vi "test_json.vi"() -> ()   [LabVIEW 2019, in "Inst.Krohn-Hite-7008.lvclass"]
uses:
  Inst.Krohn-Hite-7008.lvclass
  KH7008/typedefs/allChannelProperties--Array.ctl
  KH7008/typedefs/channelProperties--Cluster.ctl
  KH7008/typedefs/channel--enum.ctl
  KH7008/typedefs/gain--enum.ctl
  KH7008/typedefs/Input--Enum.ctl
  KH7008/typedefs/shunt--enum.ctl
  KH7008/typedefs/couple--Enum.ctl
  KH7008/typedefs/Filter--Enum.ctl
  Typedefs/setAllChannelsRequest--Cluster.ctl
  aca3e566-98a3-49c5-b33f-164d3aa1c4d2.vi
  <vilib>/JDP Science/JSONtext/Variant to JSON Text.vi
  <vilib>/addons/_JKI Toolkits/Caraya/classes/Assert/Assert Equal Value and Type_Variant.vi
  <vilib>/JDP Science/JSONtext/LVClass Serializer/JSONtext LVClass Serializer.lvclass
  KH7008/KH7008.lvlib
  <vilib>/JDP Science/JSONtext/JSONtext.lvlib
  <vilib>/addons/_JKI Toolkits/Caraya/classes/Assert/Assert.lvclass
  <vilib>/addons/_JKI Toolkits/Caraya/classes/Test/Test.lvclass
panel:
  out "allChannelProperties":T1
  in  "Channel Parameters out":T1
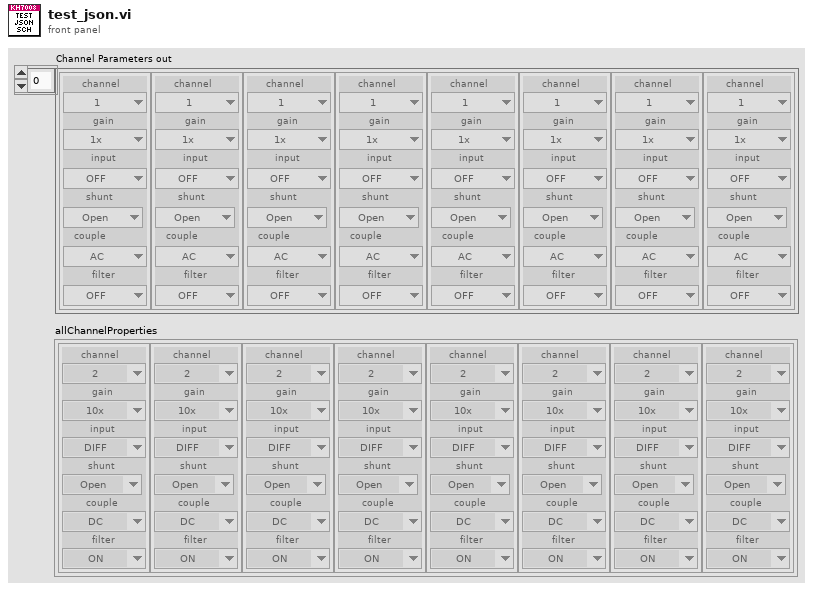
[diagram p1: front panel]
types:
  T1 = typedef "KH7008.lvlib/allChannelProperties--Array.ctl" = T2[]
  T2 = typedef "KH7008.lvlib/channelProperties--Cluster.ctl" = cluster{"channel":T3, "gain":T4, "input":T5, "shunt":T6, "couple":T7, "filter":T8}
  T3 = typedef "KH7008.lvlib/channel--enum.ctl" = enum16{"1", "2", "3", "4", "5", "6", "7", "8"}
  T4 = typedef "KH7008.lvlib/gain--enum.ctl" = enum16{"1x", "10x", "100x", "1000x"}
  T5 = typedef "KH7008.lvlib/input--enum.ctl" = enum16{"OFF", "SE+", "SE-", "DIFF"}
  T6 = typedef "KH7008.lvlib/shunt--enum.ctl" = enum16{"Open", "50", "500", "5k", "50k", "10M"}
  T7 = typedef "KH7008.lvlib/couple--enum.ctl" = enum16{"AC", "DC"}
  T8 = typedef "KH7008.lvlib/filter--enum.ctl" = enum16{"OFF", "ON"}
  T9 = typedef "Inst.Krohn-Hite-7008.lvclass/setAllChannelsRequest--Cluster.ctl" = cluster{"allChannelProperties":T1}
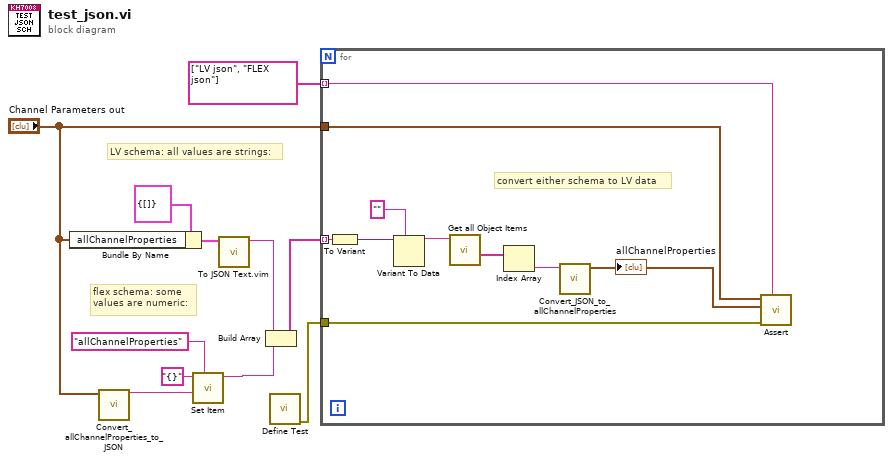
[diagram p0: block diagram]
diagram:
  # "LV schema: all values are strings:"
  # "flex schema: some\nvalues are numeric:"
  n1 = Bundle By Name(cluster=T9 {"allChannelProperties"=[]} ("setAllChannelRequest"), "allChannelProperties"="Channel Parameters out") -> (w10:T9)
  n2 = call "Convert_allChannelProperties_to_JSON.vi"("allChannelProperties"="Channel Parameters out") -> ("<JSON>"=w6:string)  [unwired: 9 in, 1 out]
  n3 = call <vilib>:"Set Item.vi"("$Path or Item Name"="allChannelProperties", "JSON to Insert"=w6, "JSON"="{}") -> ("<JSON>"=w5:string)  [unwired: 5 in, 2 out]
  n4 = call "To JSON Text.vim"("Anything"=w10) -> ("<JSON>"=w4:string)  [unwired: 9 in, 1 out]
  n5 = Build Array(w4, w5) -> (w3:string[])
  n6 = call <vilib>:"Define Test.vi"() -> ("error out"=w1:errorcluster)  [unwired: 10 in, 1 out]
  n7 = for {
    tunnel: "Channel Parameters out" -> [w15]
    tunnel: w3 -> [w14] mode=indexing
    tunnel: string[] ["LV json", "FLEX json"] ("Label") -> [w13] mode=indexing
    tunnel: w1 -> [w12]
    # "convert either schema to LV data"
    n8 = To Variant(anything=w14) -> (Variant=w17:variant)
    n9 = Variant To Data(type="", Variant=w17) -> (data=w19:string)  [unwired: 1 in, 1 out]
    n10 = call <vilib>:"Get all Object Items.vi"("JSON"=w19) -> ("<JSON>"=w21:string[])  [unwired: 7 in, 3 out]
    n11 = Index Array(array=w21) -> (element=w20:string)  [unwired: 1 in]
    n12 = call "Convert_JSON_to_allChannelProperties.vi"("<JSON>"=w20) -> ("allChannelProperties"=w16:T1)  [unwired: 9 in, 1 out]
    "allChannelProperties" <- w16
    n13 = call-poly <vilib>:"Assert.vi"("Label"=w13, "error in (no error)"=w12, "Y"=w16, "X"=w15) -> ()  [unwired: 6 in, 2 out]
  }
